vi "Boolen Array to Int FXP 12 bit.vi"(10 "Boolean array":bool[](array[boolean])) -> (0 "UNSigned":fxp<+,12,12>, 3 "Signed":fxp<+/-,12,12>)   [LabVIEW 2014]
doc: "This subVI converts a 12bit boolean array in a Signed/Unsigned 12 bit Fixed point"
panel:
  out "I16":i16
  out "U16":u16
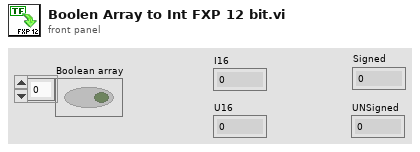
[diagram p1: front panel]
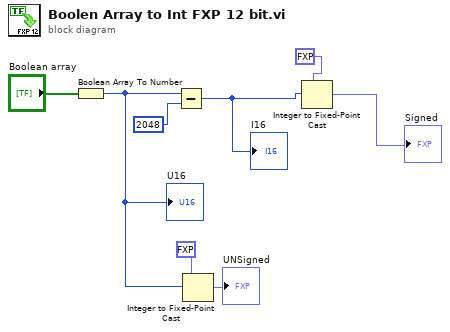
[diagram p0: block diagram]
diagram:
  n1 = Boolean Array To Number(Boolean array="Boolean array") -> (number=w4:u16)
  "U16" <- w4
  n2 = Subtract(x=w4, y=u16 2048) -> (x-y=w7:i16)
  "I16" <- w7
  n3 = Integer to Fixed-Point Cast(fixed-point type=fxp<+,12,12> 0.0, integer=w4) -> (fixed-point=→"UNSigned":fxp<+,12,12>)
  n4 = Integer to Fixed-Point Cast(fixed-point type=fxp<+/-,12,12> 0.0, integer=w7) -> (fixed-point=→"Signed":fxp<+/-,12,12>)
